vi "oa_FIR Preprocess Filter Specification Conversion.vi"(7 "filter types":T2(ring), 8 "error in":errorcluster, 10 "ripple specs [dB]":cluster{"pass band":dbl, "stop band":dbl}={"pass band"=0.1, "stop band"=60.0} {"stop band" format="%0.2f"; "pass band" format="%0.2f"}, 11 "freq specs":T1={"fpass 1"=0.125, "fstop 1"=0.45, "fpass 2"=0.125, "fstop 2"=0.45} {"fstop 2" format="%0.2f"; "fpass 2" format="%.3f"; "fstop 1" format="%0.2f"; "fpass 1" format="%.3f"}) -> (0 "error out":errorcluster, 1 "low cutoff freq: fl":dbl, 2 "high cutoff freq: fh":dbl, 3 "min transition band":dbl, 4 "A stop (dB)":dbl)   [LabVIEW 2017, in "SoundVib_RefDataProcess.lvlib"]
uses:
  <vilib>/addons/Sound and Vibration/Order Analysis/Referece Data Processing/SoundVib_RefDataProcess.lvlib
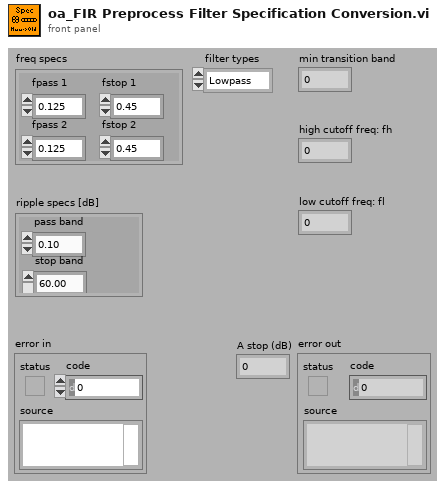
[diagram p1: front panel]
types:
  T1 = cluster{"fpass 1":dbl, "fstop 1":dbl, "fpass 2":dbl, "fstop 2":dbl}
  T2 = enum32{"Lowpass", "Highpass", "Bandpass", "Bandstop"}
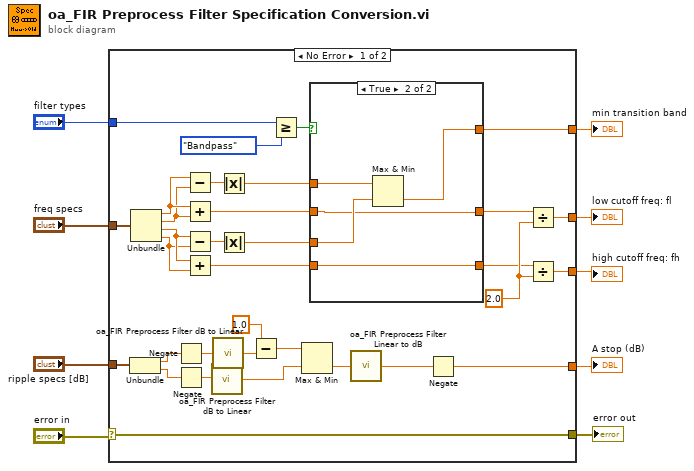
[diagram p0: block diagram]
diagram:
  n1 = case shown="No Error" "error in" {
    selector: "error in" -> [w11 w51]
    tunnel: "ripple specs [dB]" -> [w42 _]
    tunnel: "freq specs" -> [w41 _]
    tunnel: "filter types" -> [w39 _]
    tunnel: [w29 _] -> w6
    tunnel: [w23 _] -> w5
    tunnel: [w22 _] -> w4
    tunnel: [w10 _] -> w3
    tunnel: [w11 w51] -> w1
    frame No Error {
      w40 = 2.0 ("y")
      n2 = Unbundle(w42) -> ("pass band"=w21:dbl, "stop band"=w20:dbl)
      n3 = Unbundle(w41) -> ("fpass 1"=w36:dbl, "fstop 1"=w35:dbl, "fpass 2"=w34:dbl, "fstop 2"=w33:dbl)
      n4 = Negate(x=w21) -> (-x=w19:dbl)
      n5 = Negate(x=w20) -> (-x=w18:dbl)
      n6 = Subtract(x=w36, y=w35) -> (x-y=w32:dbl)
      n7 = Add(x=w36, y=w35) -> (x+y=w27:dbl)
      n8 = Subtract(x=w34, y=w33) -> (x-y=w31:dbl)
      n9 = Add(x=w34, y=w33) -> (x+y=w26:dbl)
      n10 = call <vilib>:"oa_FIR Preprocess Filter dB to Linear.vi"("dB value"=w18) -> ("linear value"=w14:dbl)
      n11 = call <vilib>:"oa_FIR Preprocess Filter dB to Linear.vi"("dB value"=w19) -> ("linear value"=w17:dbl)
      n12 = Absolute Value(x=w32) -> (abs(x)=w30:dbl)
      n13 = Absolute Value(x=w31) -> (abs(x)=w28:dbl)
      n14 = Subtract(x=1.0, y=w17) -> (x-y=w15:dbl)
      n15 = Greater Or Equal?(x=w39, y=T2."Bandpass") -> (x >= y?=w37:bool)
      n16 = Max & Min(x=w15, y=w14) -> (min(x,y)=w13:dbl)  [unwired: 1 out]
      n17 = case shown="True" w37 {
        tunnel: w30 -> [w45 w50]
        tunnel: [w45 w48] -> w29
        tunnel: w28 -> [_ w49]
        tunnel: w27 -> [w44 w47]
        tunnel: w26 -> [w43 w46]
        tunnel: [w44 w47] -> w25
        tunnel: [w43 w46] -> w24
        frame False {
        }
        frame True {
          n18 = Max & Min(x=w50, y=w49) -> (min(x,y)=w48:dbl)  [unwired: 1 out]
        }
      }
      n19 = call <vilib>:"oa_FIR Preprocess Filter Linear to dB.vi"("linear value"=w13) -> ("dB value"=w12:dbl)
      n20 = Negate(x=w12) -> (-x=w10:dbl)
      n21 = Divide(x=w25, y=w40) -> (x/y=w22:dbl)
      n22 = Divide(x=w24, y=w40) -> (x/y=w23:dbl)
    }
    frame Error {
    }
  }
  "high cutoff freq: fh" <- w5
  "low cutoff freq: fl" <- w4
  "A stop (dB)" <- w3
  "min transition band" <- w6
  "error out" <- w1
